vi "proc_flush_stdout.vi"(7 "interval [ms]":i32=100, 8 "error in":errorcluster, 11 "process instance handle in":u32[](array[numeric])) -> (0 "error out":errorcluster, 2 "exited":bool, 3 "process instance handle out":u32[](array[numeric]))   [LabVIEW 2011]
doc: "Flushes stdout pipe data. Time interval is maximum interval between successive data block from process instance."
panel:
  in  "exit mem":i32
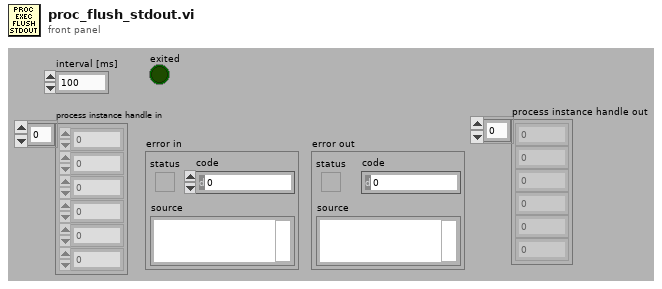
[diagram p1: front panel]
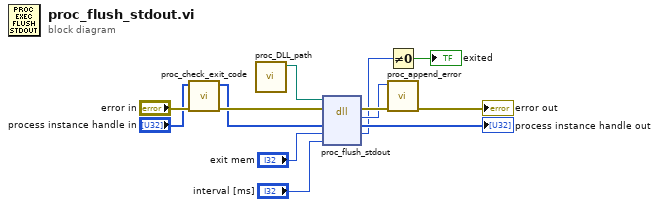
[diagram p0: block diagram]
diagram:
  n1 = call "proc_check_exit_code.vi"("error in"="error in", "instance handle in"="process instance handle in") -> ("error out"=w3:errorcluster, "instance handle out"=w1:u32[])  [unwired: 5 in, 3 out]
  n2 = call "proc_DLL_path.vi"() -> ("path out"=w13:path)  [unwired: 10 in, 1 out]
  n3 = dll-call lib="lv_proc.dll" fn="proc_flush_stdout"(path in=w13, error in=w3, "proc"=w1, "exit"="exit mem", "interval"="interval [ms]") -> (error out=w11:errorcluster, "error"=w10:i32, "proc"=→"process instance handle out":u32[], "exit"=w7:i32)  [unwired: 2 in, 1 out]
  n4 = Not Equal To 0?(x=w7) -> (x != 0?=→"exited":bool)
  n5 = call "proc_append_error.vi"("error in"=w11, "code in"=w10) -> ("error out"=→"error out":errorcluster)  [unwired: 8 in, 1 out]
